vi "sent by focus stage QM.vi"(8 "error in (no error)":errorcluster, 10 "ProceedMessage":refnum<class "ProceedMessage.lvclass">, 11 "Autofocus in":refnum<class "Autofocus.lvclass">) -> (0 "error out":errorcluster, 1 "sent by focus stage?":bool, 2 "ProceedMessage 2":refnum<class "ProceedMessage.lvclass">, 3 "Autofocus out":refnum<class "Autofocus.lvclass">)   [LabVIEW 2012, in "Autofocus.lvclass"]
uses:
  Autofocus.lvclass
  <vilib>/Distrio/Murmex/ProceedMessage/ProceedMessage.lvclass
  Autofocus.lvclass/Autofocus.ctl
  <vilib>/Distrio/Murmex/Message/Message.lvclass
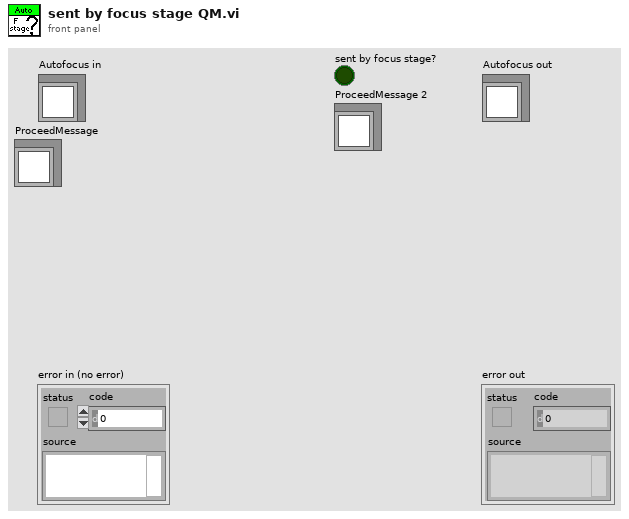
[diagram p1: front panel]
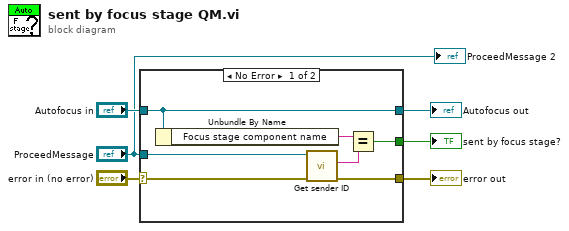
[diagram p0: block diagram]
diagram:
  n1 = case shown="No Error" "error in (no error)" {
    selector: "error in (no error)" -> [w9 w15]
    tunnel: [w8 w15] -> w5
    tunnel: [w11 w14] -> w3
    tunnel: "Autofocus in" -> [w11 w14]
    tunnel: [w10 _] -> w2
    tunnel: "ProceedMessage" -> [w7 _]
    frame No Error {
      n2 = Unbundle By Name(w11) -> ("Focus stage component name"=w12:string)
      n3 = call <vilib>:"Get sender ID.vi"("error in (no error)"=w9, "Message in"=w7) -> ("error out"=w8:errorcluster, "sender"=w13:string)  [unwired: 7 in, 1 out]
      n4 = Equal?(x=w12, y=w13) -> (x = y?=w10:bool)
    }
    frame Error {
    }
  }
  "error out" <- w5
  "Autofocus out" <- w3
  "sent by focus stage?" <- w2
  "ProceedMessage 2" <- "ProceedMessage"
